vi "publishWavelength.vi"(8 "error in (no error)":errorcluster, 10 "wavelength":T1, 11 "MonoCommunicator in":refnum<class "MonoCommunicator.lvclass">) -> (0 "error out":errorcluster, 3 "MonoCommunicator out":refnum<class "MonoCommunicator.lvclass">)   [LabVIEW 2016, in "MonoCommunicator.lvclass"]
uses:
  MonoCommunicator.lvclass
  Typedefs/wavelength.ctl
  Typedefs/publishers.ctl
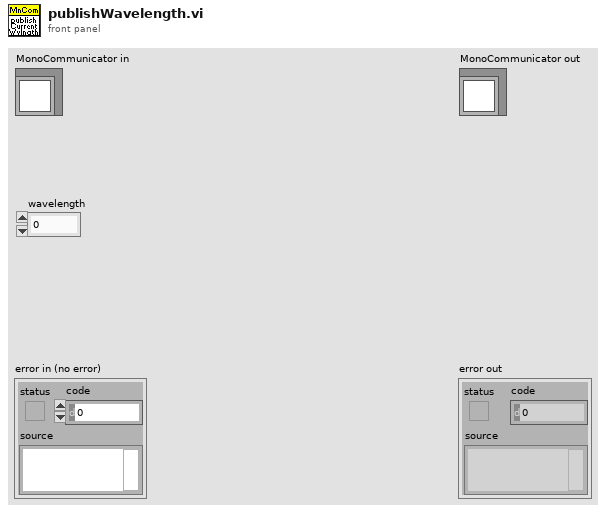
[diagram p1: front panel]
types:
  T1 = typedef "wavelength.ctl" = dbl
  T2 = typedef "publishers.ctl" = enum16{"Wavelength", "Grating", "FrontEntranceSlitPosition", "FrontExitSlitPosition", "SoftwareStatus", "MonochromatorId"}
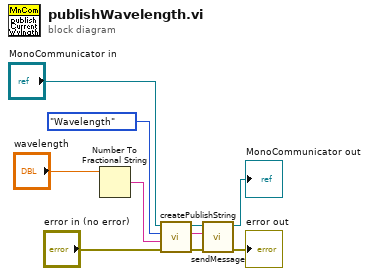
[diagram p0: block diagram]
diagram:
  n1 = Number To Fractional String(number="wavelength") -> (F-format string=w1:string)  [unwired: 3 in]
  n2 = call "createPublishString.vi"("error in (no error)"="error in (no error)", "parameter"=w1, "publishers"=publishers."Wavelength", "MonoCommunicator in"="MonoCommunicator in") -> ("error out"=w5:errorcluster, "string"=w6:string, "MonoCommunicator out"=w7:refnum<class "MonoCommunicator.lvclass">)  [unwired: 5 in]
  n3 = call "sendMessage.vi"("error in (no error)"=w5, "message"=w6, "MonoCommunicator in"=w7) -> ("error out"=→"error out":errorcluster, "MonoCommunicator out"=→"MonoCommunicator out":refnum<class "MonoCommunicator.lvclass">)  [unwired: 7 in]
